vi "Generate Reports.vi"(0 "target dir":path=path "C:/ADIBitbucket/nists19.0_templateproject/Code Modules/Common/Instrument Control", 5 "output file(s) path":path=path "../docs", 11 "error in":errorcluster) -> (15 "error out":errorcluster={"status"=TRUE, "code"=118, "source"="Invoke Node in VI Documenation MD Report Gen.lvlib:Format VI Information.vi:2500001->VI Documenation MD Report Gen.lvlib:Generate Documentation from VIs.vi->VI Documenation MD Report Gen.lvlib:Auto Generate Reports.vi\n<APPEND>\nMethod Name: <b>Print:VI To HTML</b>"})   [LabVIEW 2019, in "MD Generator.lvlib"]
uses:
  MD Generator.lvlib
  subVIs/Report Path Cluster.ctl
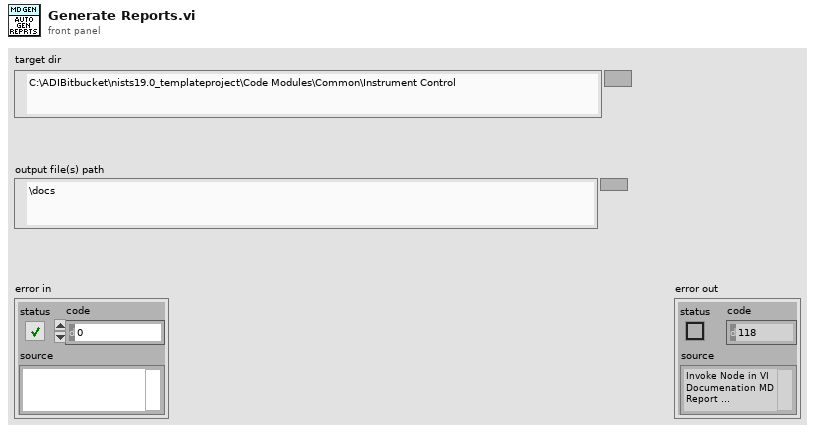
[diagram p1: front panel]
types:
  T1 = typedef "MD Generator.lvlib/Report Path Cluster.ctl" = cluster{"target dir":path, "current dir":path, "output dir":cluster{"base dir":path, "image dir":path, "html dir":path, "md dir":path}, "folder names":string[], "filenames":string[]}
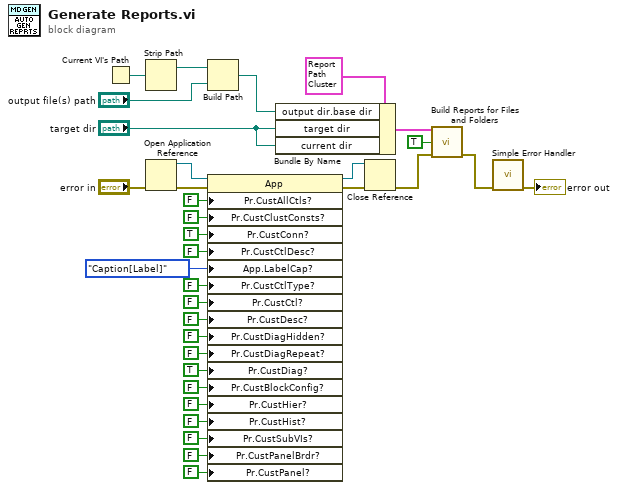
[diagram p0: block diagram]
diagram:
  n1 = Current VI's Path() -> (path=w31:path)
  n2 = Strip Path(path=w31) -> (stripped path=w30:path)  [unwired: 1 out]
  n3 = Open Application Reference(8:"error in") -> (0:w23:errorcluster, 3:w4:refnum<vi>)  [unwired: 3 in]
  n4 = Build Path(base path=w30, name or relative path="output file(s) path") -> (appended path=w25:path)
  n5 = property on="Property Node" class="App"(reference=w4, error in=w23, "Pr.CustAllCtls?"=FALSE ("Printing:Custom All Controls?"), "Pr.CustClustConsts?"=FALSE ("Printing:Custom Cluster Constants?"), "Pr.CustConn?"=TRUE ("Printing:Custom Connector?"), "Pr.CustCtlDesc?"=FALSE ("Printing:Custom Control Descriptions?"), "App.LabelCap?"=enum16{"Label", "Caption", "Caption[Label]"}."Caption[Label]" ("Printing:Custom Control Label/Caption?"), "Pr.CustCtlType?"=FALSE ("Printing:Custom Control Types?"), "Pr.CustCtl?"=FALSE ("Printing:Custom Controls?"), "Pr.CustDesc?"=FALSE ("Printing:Custom Description?"), "Pr.CustDiagHidden?"=FALSE ("Printing:Custom Diagram Hidden?"), "Pr.CustDiagRepeat?"=FALSE ("Printing:Custom Diagram Repeat?"), "Pr.CustDiag?"=TRUE ("Printing:Custom Diagram?"), "Pr.CustBlockConfig?"=FALSE ("Printing:Custom Express VI Configuration?"), "Pr.CustHier?"=FALSE ("Printing:Custom Hierarchy?"), "Pr.CustHist?"=FALSE ("Printing:Custom History?"), "Pr.CustSubVIs?"=FALSE ("Printing:Custom List of SubVIs?"), "Pr.CustPanelBrdr?"=FALSE ("Printing:Custom Panel Border?"), "Pr.CustPanel?"=FALSE ("Printing:Custom Panel?")) -> (reference out=w3:refnum<vi>, error out=w22:errorcluster)
  n6 = Bundle By Name(cluster=T1 {"target dir"=path "C:/ADIBitbucket/nists19.0_templateproject/Code Modules/Common/Instrument Control/DCPower", "current dir"=path "C:/ADIBitbucket/nists19.0_templateproject/Code Modules/Common/Instrument Control/DCPower", "output dir"={"base dir"=path "../docs", "image dir"=path "../docs", "html dir"=path "../docs", "md dir"=path "../docs"}, "folder names"=[], "filenames"=[]} ("directory info in"), "output dir.base dir"=w25, "target dir"="target dir", "current dir"="target dir") -> (w27:T1)
  n7 = Close Reference(reference=w3, error in (no error)=w22) -> (error out=w26:errorcluster)
  n8 = call "Build Reports for Files and Folders.vi"("directory info"=w27, "Initial Call"=TRUE, "error in"=w26) -> ("error out"=w24:errorcluster)  [unwired: 12 in]
  n9 = call <vilib>:"Simple Error Handler.vi"("error in (no error)"=w24) -> ("error out"=→"error out":errorcluster)  [unwired: 4 in, 4 out]
